vi "LVDimInterface.dis_add_command_notifier.vi"(1 "notifier":T1, 3 "commandName":string, 4 "typeDescriptor":string, 5 "error in (no error)":errorcluster) -> (14 "commandID":i32, 19 "error out":errorcluster)   [LabVIEW 2013, in "LVDimInterface.lvlib"]
doc: "Add a command to a DIM server. Whenever a new command is received by the server, the command data will be inserted into the LabVIEW event structure specified.\n\nImportant: One must call \"start serving\" to declare the new service to the dim name server.\n\nHistory: 16-DEC-2005, Dietrich Beck\n\nCopyright (C)\nGesellschaft für Schwerionenforschung, GSI\nPlanckstr. 1\n64291 Darmstadt\nGermany\n\nContact: D.Beck@gsi.de \n\nThis program is free software; you can redistribute it and/or modify it under the terms of the \nGNU General Public License as published by the Free Software Foundation; either version 2 of the license, or (at your option) any later version.\n\nThis program is distributed in the hope that it will be useful, but WITHOUT ANY WARRANTY; without even the implied warranty of MERCHANTABILITY or FITNESS FOR A PARTICULAR PURPOSE. See the GNU General License for more details (http://www.gnu.org).\n\nGesellschaft für Schwerionenforschung, GSI\nPlanckstr. 1, 64291 Darmstadt, Germany\nFor all questions and ideas contact D. Beck.\nLast update: 16-DEC-2005"
uses:
  LVDimInterface.lvlib
  LVDimInterface.notifier type.ctl
  bin/libDimWrapper.dll
  C/GPL/Projects/DimLVEvent/bin/libDimWrapper.so
  C/GPL/Projects/DimLVEvent/bin/libDimWrapperSPL.dll
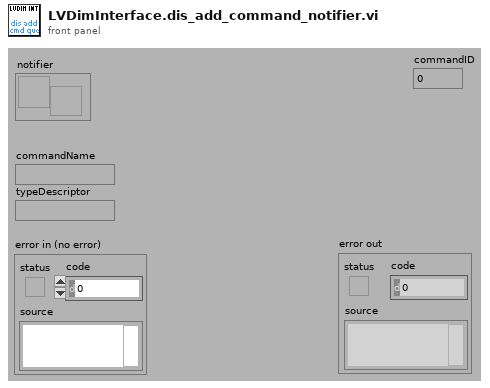
[diagram p1: front panel]
types:
  T1 = typedef "LVDimInterface.lvlib/LVDimInterface.notifier type.ctl" = refnum<notifier>
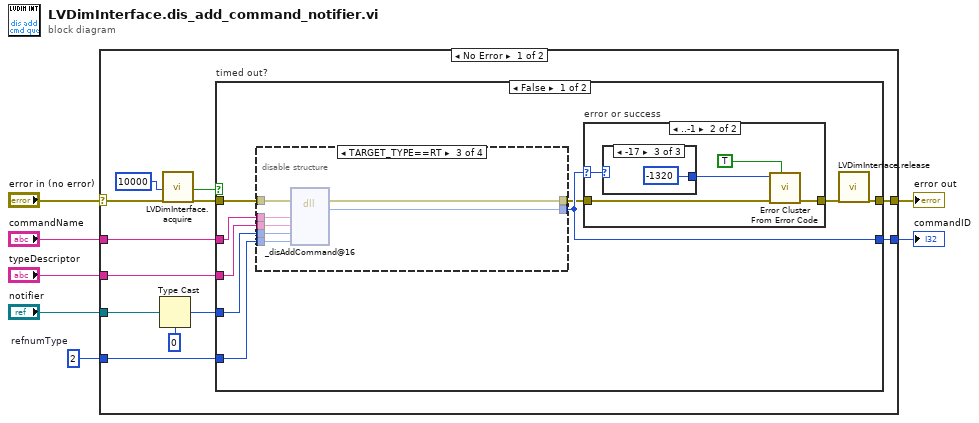
[diagram p0: block diagram]
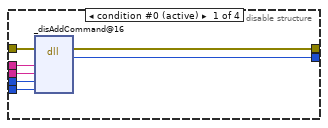
[diagram p2: hidden frame]
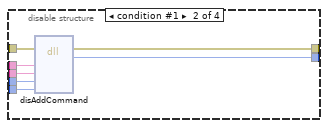
[diagram p3: hidden frame]
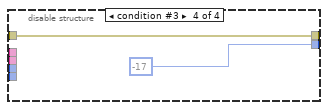
[diagram p4: hidden frame]
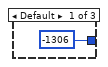
[diagram p6: hidden frame]
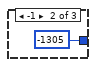
[diagram p7: hidden frame]
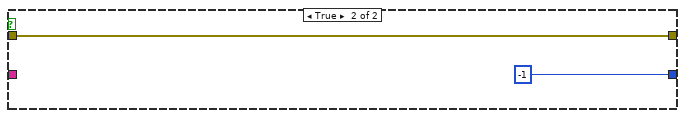
[diagram p8: hidden frame]
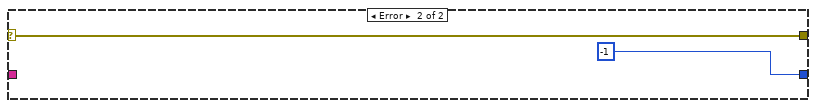
[diagram p9: hidden frame]
diagram:
  w7 = 2  # refnumType
  n1 = case shown="No Error" "error in (no error)" {
    selector: "error in (no error)" -> [w8 w63]
    tunnel: "notifier" -> [w15 _]
    tunnel: w7 -> [w16 _]
    tunnel: "commandName" -> [w19 _]
    tunnel: [w17 -1 ("commandID")] -> w5
    tunnel: [w18 w63] -> w4
    tunnel: "typeDescriptor" -> [w14 _]
    frame No Error {
      n2 = Type Cast(type=u32 0, x=w15) -> (*(type *) &x=w13:u32)
      n3 = call "LVDimInterface.acquire.vi"("ms timeout (10000)"=10000 ("ms timeout (-1)"), "error in (no error)"=w8) -> ("timed out"=w9:bool, "error out"=w11:errorcluster)  [unwired: 16 in]
      n4 = case "timed out?" shown="False" w9 {
        tunnel: w19 -> [w28 _]
        tunnel: [w20 w62] -> w18
        tunnel: [w27 -1 ("commandID")] -> w17
        tunnel: w16 -> [w26 _]
        tunnel: w13 -> [w25 _]
        tunnel: w14 -> [w24 _]
        tunnel: w11 -> [w23 w62]
        frame False {
          n5 = disable-structure "Conditional Disable Structure" shown="TARGET_TYPE==RT" {
            disable-tunnel: w28 -> [w35 w42 w49 _]
            disable-tunnel: [w34 w41 w48 -17 ("commandID")] -> w27
            disable-tunnel: w26 -> [w33 w40 w47 _]
            disable-tunnel: w25 -> [w32 w39 w46 _]
            disable-tunnel: w24 -> [w31 w38 w45 _]
            disable-tunnel: w23 -> [w30 w37 w44 w50]
            disable-tunnel: [w29 w36 w43 w50] -> w22
            frame condition #0 (active) {
              n6 = dll-call lib="C:/User/Brand/LVP/Submodules/DimLVEvent/bin/libDimWrapper.dll" fn="_disAddCommand@16"(error in=w30, "commandName"=w35, "typeDescriptor"=w31, "queueRef"=w32, "refnumType"=w33) -> (error out=w29:errorcluster, "commandID"=w34:i32)  [unwired: 6 in, 1 out]
            }
            frame condition #1 {
              n7 = dll-call lib="F:/LVSCC/C/GPL/Projects/DimLVEvent/bin/libDimWrapper.so" fn="disAddCommand" label="libDimWrapper.dll:_disAddCommand@16"(error in=w37, "commandName"=w42, "typeDescriptor"=w38, "queueRef"=w39, "refnumType"=w40) -> (error out=w36:errorcluster, "commandID"=w41:i32)  [unwired: 6 in, 1 out]
            }
            frame condition #2 {
              n8 = dll-call lib="C:/User/Brand/SVN/C/GPL/Projects/DimLVEvent/bin/libDimWrapperSPL.dll" fn="_disAddCommand@16"(error in=w44, "commandName"=w49, "typeDescriptor"=w45, "queueRef"=w46, "refnumType"=w47) -> (error out=w43:errorcluster, "commandID"=w48:i32)  [unwired: 6 in, 1 out]
            }
            frame condition #3 {
            }
          }
          n9 = case "error or success" shown="..-1" w27 {
            selector: w27 -> [_ w57]
            tunnel: w22 -> [w52 w55]
            tunnel: [w52 w56] -> w21
            frame 0, Default {
            }
            frame ..-1 {
              n10 = case shown="-17" w57 {
                tunnel: [-1306 ("f") -1305 ("code") -1320 ("code")] -> w53
                frame Default {
                }
                frame -1 {
                }
                frame -17 {
                }
              }
              n11 = call <vilib>:"Error Cluster From Error Code.vi"("show call chain? (False)"=TRUE ("status"), "error in (no error)"=w55, "error code (0)"=w53) -> ("error out"=w56:errorcluster)  [unwired: 6 in]
            }
          }
          n12 = call "LVDimInterface.release.vi"("error in (no error)"=w21) -> ("error out"=w20:errorcluster)  [unwired: 18 in]
        }
        frame True {
        }
      }
    }
    frame Error {
    }
  }
  "commandID" <- w5
  "error out" <- w4
